vi "Update Display.vi"(0 "eye scan in":refnum<class "niHighSpeedSerial Eye Scan v1 Host.lvclass">, 5 "instance":u8, 7 "IntGraph refnum":refnum<vi>, 11 "error in":errorcluster) -> (4 "eye scan out":refnum<class "niHighSpeedSerial Eye Scan v1 Host.lvclass">, 15 "error out":errorcluster)   [LabVIEW 2015, in "niHighSpeedSerial Eye Scan v1 Host.lvclass"]
doc: "Updates the X, Y, and Z scales of the passed in Intensity Graph based on the specified instance's configuration.\nThe Z scale is formatted based on the configured BER floor.\n\n<B>Input Parameters</B>\n\n<B>eye scan in</B> Takes in a reference to your session from the previous VI.\n\n<B>instance</B> The instance of the channel to be used.\n\n<B>IntGraph refnum</B> is a refnum to the Intensity Graph to be updated.\n\n<B>error in</B> describes error conditions that occur before this node runs. This input provides standard 'error in' functionality.\n\n<B>Output Parameters</B>\n\n<B>eye scan out</B> passes a reference to your session to the next VI.\n\n<B>error out</B> contains error information. This output provides standard 'error out' functionality."
uses:
  <instrlib>/niHighSpeedSerial/Eye Scan/v1/Host/Eye Scan/niHighSpeedSerial Eye Scan v1 Host.lvclass
  <instrlib>/niHighSpeedSerial/Eye Scan/v1/Host/Eye Scan/niHighSpeedSerial Eye Scan v1 Host.lvclass/niHighSpeedSerial Eye Scan v1 Host.ctl
  <vilib>/Utility/miscctls.llb/LVFormatAndPrecisionTypeDef.ctl
  <instrlib>/niHighSpeedSerial/Eye Scan/v1/Host/Impl/Eye Scan Point Iterator/niHighSpeedSerial Eye Scan Point Iterator v1 Host.lvclass
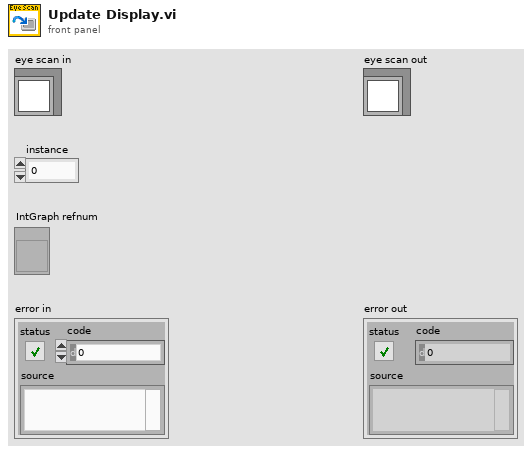
[diagram p1: front panel]
types:
  T1 = typedef "LVFormatAndPrecisionTypeDef.ctl" = cluster{"Format":u8, "Precision":u8}
  T2 = typedef "niHighSpeedSerial Eye Scan v1 Host.lvclass/Private Data.ctl" = cluster{"instruction target":refnum<class "niInstr Instruction Target v1 Host.lvclass">, "channels":T3[], "measure state":T4, "rx output divider":T5, "equalization mode":T6, "rx data width":T7, "BER floor":dbl, "number of points completed":i32, "rx output divider configured?":bool, "equalization mode configured?":bool, "rx data width configured?":bool}
  T3 = typedef "niHighSpeedSerial Eye Scan v1 Host.lvclass/Channel Data.ctl" = cluster{"instance":u8, "channel":refnum<class "niHighSpeedSerial Eye Scan Single Point v1 Host.lvclass">, "point iterator":refnum<class "niHighSpeedSerial Eye Scan Point Iterator v1 Host.lvclass">}
  T4 = typedef "niHighSpeedSerial Eye Scan v1 Host.lvclass/Measure State.ctl" = enum16{"Uninitialized", "Initialized", "Ready", "Measuring", "Finished", "Aborted"}
  T5 = typedef "niHighSpeedSerial Eye Scan Common v1 Host.lvlib/RX Output Divider.ctl" = enum16{"1", "2", "4", "8", "16"}
  T6 = typedef "niHighSpeedSerial Eye Scan Common v1 Host.lvlib/Equalization Mode.ctl" = enum16{"DFE", "LPM"}
  T7 = typedef "niHighSpeedSerial Eye Scan Common v1 Host.lvlib/Data Width.ctl" = enum16{"16 Bit", "20 Bit", "32 Bit", "40 Bit"}
  T8 = typedef "LVRangeTypeDef.ctl" = cluster{"Minimum":dbl, "Maximum":dbl, "Increment":dbl, "Minor Increment":dbl, "Start":dbl}
  T9 = typedef "LVOffsetAndMultiplierTypeDef.ctl" = cluster{"Offset":dbl, "Multiplier":dbl}
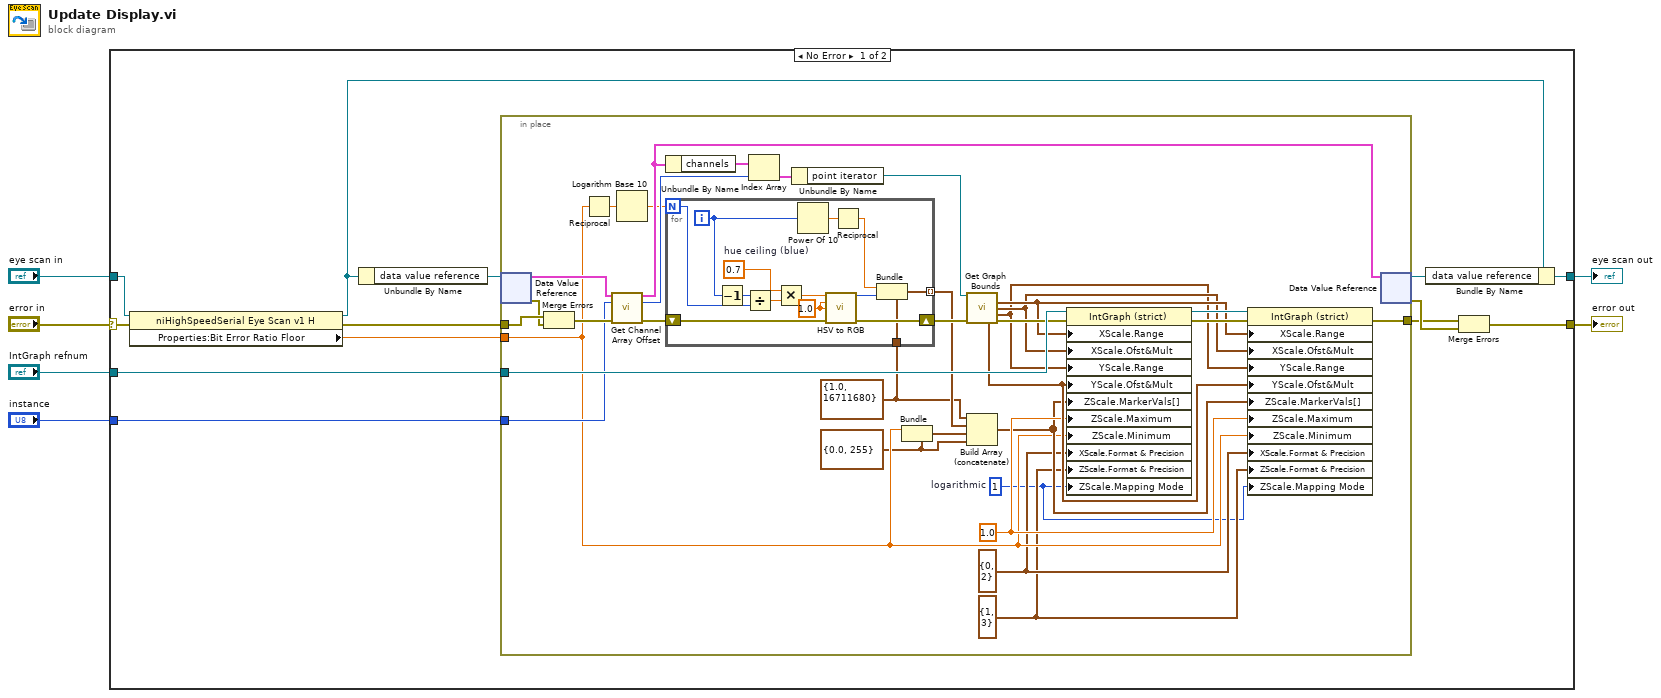
[diagram p0: block diagram]
diagram:
  n1 = case shown="No Error" "error in" {
    selector: "error in" -> [w9 w68]
    tunnel: [w15 w68] -> w5
    tunnel: "IntGraph refnum" -> [w19 _]
    tunnel: [w16 w67] -> w2
    tunnel: "eye scan in" -> [w11 w67]
    tunnel: "instance" -> [w12 _]
    frame No Error {
      n2 = property class="niHighSpeedSerial Eye Scan v1 H"(reference=w11, error in=w9) -> (reference out=w10:refnum<class "niHighSpeedSerial Eye Scan v1 Host.lvclass">, error out=w8:errorcluster, "Properties:Bit Error Ratio Floor"=w7:dbl)
      n3 = Unbundle By Name(w10) -> ("data value reference"=w18:refnum<data-value>)
      n4 = in-place {
        in-place-border: w19 -> [w52]
        in-place-border: w8 -> [w51]
        in-place-border: [w43] -> w13
        in-place-border: w12 -> [w32]
        in-place-border: w7 -> [w29]
        w20 = u8 1  # logarithmic
        w25 = T1 {"Format"=1, "Precision"=3} ("Z Scale.Display Format")
        w26 = T1 {"Format"=0, "Precision"=2} ("X Scale.Display Format")
        w21 = cluster{dbl, u32} {1.0, 16711680}
        w24 = cluster{dbl, u32} {0.0, 255}
        w38 = 1.0 ("Z Scale.Range:Maximum")
        n5 = in-place-dvr #1(w18) -> (w34:T2, w50:errorcluster)
        n6 = Merge Errors(w51, w50) -> (w35:errorcluster)
        n7 = Reciprocal(x=w29) -> (1/x=w36:dbl)
        n8 = call <instrlib>:"Get Channel Array Offset.vi"("private data"=w34, "instance"=w32, "error in"=w35) -> ("private data out"=w33:T2, "channel array offset"=w31:i32, "error out"=w28:errorcluster)  [unwired: 10 in]
        n9 = Logarithm Base 10(1:w36) -> (0:w30:dbl)
        n10 = Unbundle By Name(w33) -> ("channels"=w49:T3[])
        n11 = for {
          N: w30 -> [w66]
          tunnel: [w59] -> w23 mode=indexing
          shift-right: [w57] -> w27
          shift-left: w28 -> [w58]
          tunnel: w21 -> [w53]
          i -> [w62]
          w54 = 0.7  # hue ceiling (blue)
          w64 = 1.0 ("Value")
          n12 = Decrement(x=w62) -> (x-1=w56:i32)
          n13 = Divide(x=w56, y=w66) -> (x/y=w65:dbl)
          n14 = Multiply(x=w54, y=w65) -> (x*y=w55:dbl)
          n15 = Power Of 10(x=w62) -> (10^x=w63:dbl)
          n16 = call <instrlib>:"HSV to RGB.vi"("Hue"=w55, "Saturation"=w64, "Value"=w64, "error in"=w58) -> ("Color"=w61:u32, "error out"=w57:errorcluster)  [unwired: 10 in]
          n17 = Reciprocal(x=w63) -> (1/x=w60:dbl)
          n18 = Bundle(cluster=w53, w60, w61) -> (w59:cluster{dbl, u32})
        }
        n19 = Index Array(array=w49, index=w31) -> (element=w48:T3)
        n20 = Unbundle By Name(w48) -> ("point iterator"=w47:refnum<class "niHighSpeedSerial Eye Scan Point Iterator v1 Host.lvclass">)
        n21 = Bundle(cluster=w24, w29) -> (w22:cluster{dbl, u32})  [unwired: 1 in]
        n22 = call-dynamic "Get Graph Bounds.vi"("eye scan point iterator"=w47, "error in"=w27) -> ("x scale.range"=w42:T8, "x scale.offset and multiplier"=w41:T9, "y scale.range"=w40:T8, "y scale.offset and multiplier"=w39:T9, "error out"=w46:errorcluster)  [unwired: 8 in, 1 out]
        n23 = Build Array (concatenate)(w21, w23, w22, w24) -> (w37:cluster{dbl, u32}[])
        n24 = property class="IntGraph (strict)"(reference=w52, error in=w46, "XScale.Range"=w42, "XScale.Ofst&Mult"=w41, "YScale.Range"=w40, "YScale.Ofst&Mult"=w39, "ZScale.MarkerVals[]"=w37, "ZScale.Maximum"=w38, "ZScale.Minimum"=w29, "XScale.Format & Precision"=w26, "ZScale.Format & Precision"=w25, "ZScale.Mapping Mode"=w20) -> (reference out=w45:refnum<vi>, error out=w44:errorcluster)
        n25 = property class="IntGraph (strict)"(reference=w45, error in=w44, "XScale.Range"=w42, "XScale.Ofst&Mult"=w41, "YScale.Range"=w40, "YScale.Ofst&Mult"=w39, "ZScale.MarkerVals[]"=w37, "ZScale.Maximum"=w38, "ZScale.Minimum"=w29, "XScale.Format & Precision"=w26, "ZScale.Format & Precision"=w25, "ZScale.Mapping Mode"=w20) -> (error out=w43:errorcluster)  [unwired: 1 out]
        n26 = in-place-dvr #1(w33) -> (w17:refnum<data-value>, w14:errorcluster)
      }
      n27 = Bundle By Name(cluster=w10, "data value reference"=w17) -> (w16:refnum<class "niHighSpeedSerial Eye Scan v1 Host.lvclass">)
      n28 = Merge Errors(w13, w14) -> (w15:errorcluster)
    }
    frame Error {
    }
  }
  "error out" <- w5
  "eye scan out" <- w2
